vi "004 Array superior a u.vi"() -> ()   [LabVIEW 2019]
panel:
  out "Array":bool[](array[boolean])
  out "Random array":dbl[](array[numeric])
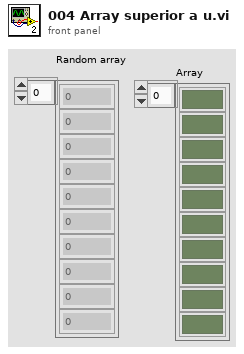
[diagram p1: front panel]
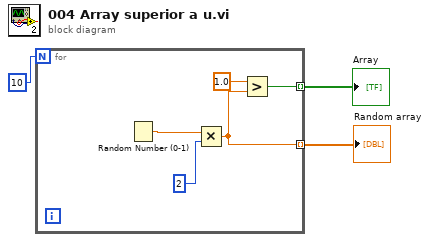
[diagram p0: block diagram]
diagram:
  n1 = for {
    N: 10 -> [_]
    tunnel: [w5] -> w2 mode=indexing
    tunnel: [w4] -> w1 mode=indexing
    n2 = Random Number (0-1)() -> (number: 0 to 1=w8:dbl)
    n3 = Multiply(x=w8, y=2) -> (x*y=w4:dbl)
    n4 = Greater?(x=1.0, y=w4) -> (0:w5:bool)
  }
  "Random array" <- w1
  "Array" <- w2
